vi "Calculate Directions.vi"(8 "error in (no error)":errorcluster, 10 "Heading":T1=enum."Right", 11 "Grassfire in":refnum<class "Grassfire.lvclass">) -> (0 "error out":errorcluster, 2 "Directions":T1[](array[typedef]), 3 "Grassfire out":refnum<class "Grassfire.lvclass">)   [LabVIEW 2019, in "Grassfire.lvclass"]
uses:
  Grassfire.lvclass
  Direction--enum.ctl
  Address/Address.lvclass
  Grassfire.lvclass/Grassfire.ctl
  Node/Node Value.lvclass/Node Value.ctl
  Node/Node Type--enum.ctl
  <userlib>/_OpenG.lib/array/array.llb/Sort 1D Array (I32)__ogtk.vi
  <userlib>/_OpenG.lib/array/array.llb/Reorder 1D Array2 (I16)__ogtk.vi
  Node/Node Value.lvclass
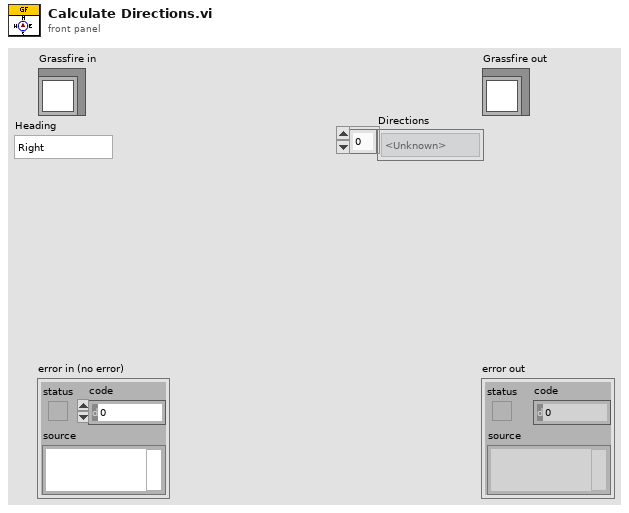
[diagram p1: front panel]
types:
  T1 = typedef "Grassfire.lvclass/Direction--enum.ctl" = enum16{"<Unknown>", "Right", "Down", "Left", "Up"}
  T2 = map{refnum<class "Address.lvclass">, refnum<class "Node Value.lvclass">}
  T3 = typedef "Node Value.lvclass/Node Type--enum.ctl" = enum16{"Empty", "Blocked", "Start", "End", "Path"}
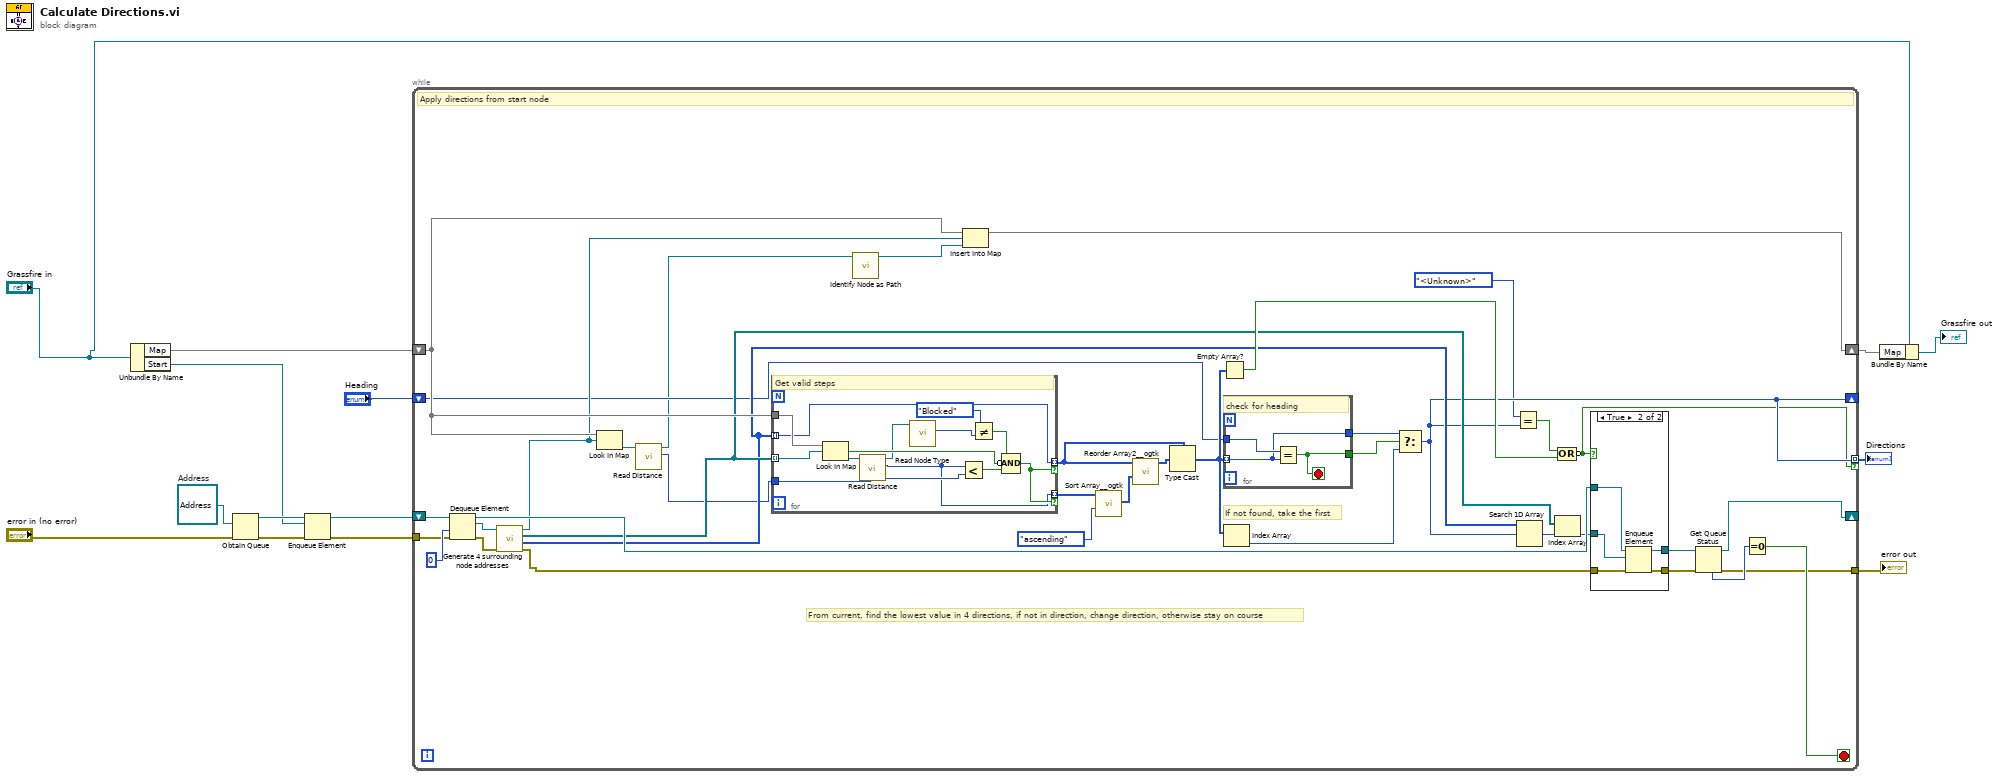
[diagram p0: block diagram]
diagram:
  w1 = refnum<class "Address.lvclass"> refnum  # Address
  n1 = Unbundle By Name("Grassfire in") -> ("Map"=w11:T2, "Start"=w10:refnum<class "Address.lvclass">)
  n2 = Obtain Queue(element data type=w1, error in (no error)="error in (no error)") -> (queue out=w13:refnum<queue>, error out=w14:errorcluster)  [unwired: 3 in, 1 out]
  n3 = Enqueue Element(queue=w13, element=w10, error in (no error)=w14) -> (queue out=w9:refnum<queue>, error out=w8:errorcluster)  [unwired: 1 in, 1 out]
  n4 = while {
    shift-right: [w48] -> w5
    shift-left: w11 -> [w49]
    shift-right: [w47] -> _
    shift-left: w9 -> [w51]
    tunnel: w8 -> [w52]
    tunnel: [w29] -> w7
    shift-right: [w17] -> _
    shift-left: "Heading" -> [w24]
    tunnel: [w17] -> w2 mode=indexing if=w16
    stop <- w46 stop-if-true
    # "If not found, take the first"
    # "From current, find the lowest value in 4 directions, if not in direction, change direction, otherwise stay on course"
    # "Apply directions from start node"
    n5 = Dequeue Element(queue=w51, timeout in ms (-1)=0, error in (no error)=w52) -> (queue out=w50:refnum<queue>, element=w28:refnum<class "Address.lvclass">, error out=w23:errorcluster)  [unwired: 1 out]
    n6 = call "Generate 4 surrounding node addresses.vi"("error in (no error)"=w23, "2D Array in"=w28) -> ("error out"=w22:errorcluster, "Search Directions"=w26:T1[], "4 Surrounding Nodes"=w27:refnum<class "Address.lvclass">[], "2D Array out"=w25:refnum<class "Address.lvclass">)  [unwired: 6 in]
    n7 = Look In Map(map=w49, key=w25) -> (value=w20:refnum<class "Node Value.lvclass">)  [unwired: 1 in, 1 out]
    n8 = call "Read Distance.vi"("Picture Ring in"=w20) -> ("Distance"=w18:i32, "Picture Ring out"=w19:refnum<class "Node Value.lvclass">)  [unwired: 8 in, 1 out]
    n9 = for {
      tunnel: w49 -> [w76]
      tunnel: w27 -> [w75] mode=indexing
      tunnel: [w69] -> w44 mode=indexing if=w73
      tunnel: [w74] -> w40 mode=indexing if=w73
      tunnel: w26 -> [w74] mode=indexing
      tunnel: w18 -> [w71]
      # "Get valid steps"
      n10 = Look In Map(map=w76, key=w75) -> (key not found?=w68:bool, value=w70:refnum<class "Node Value.lvclass">)  [unwired: 1 in]
      n11 = call "Read Distance.vi"("Picture Ring in"=w70) -> ("Distance"=w69:i32, "Picture Ring out"=w67:refnum<class "Node Value.lvclass">)  [unwired: 8 in, 1 out]
      n12 = call "Read Node Type.vi"("Picture Ring in"=w67) -> ("Node Type"=w65:T3)  [unwired: 8 in, 2 out]
      n13 = Less?(x=w69, y=w71) -> (x < y?=w72:bool)
      n14 = Not Equal?(x=Node_Type--enum."Blocked" ("Node Type"), y=w65) -> (x != y?=w64:bool)
      n15 = Compound Arithmetic op=AND(w64, invert w68, w72) -> (w73:bool)
    }
    n16 = call "Identify Node as Path.vi"("Picture Ring in"=w19) -> ("Picture Ring out"=w21:refnum<class "Node Value.lvclass">)  [unwired: 9 in, 1 out]
    n17 = Insert Into Map(map in=w49, key=w25, value=w21) -> (map out=w48:T2)  [unwired: 2 out]
    n18 = call-poly <userlib>:"Sort Array__ogtk.vi"("Order"=enum16{"ascending", "descending"}."ascending", "Array in"=w44) -> ("Sorted Pointers"=w42:i32[])  [unwired: 8 in, 1 out]
    n19 = call-poly <userlib>:"Reorder Array2__ogtk.vi"("indices"=w42, "array"=w40) -> ("reordered array"=w41:i16[])  [unwired: 9 in]
    n20 = Type Cast(type=w40, x=w41) -> (*(type *) &x=w32:T1[])
    n21 = Empty Array?(array=w32) -> (empty?=w38:bool)
    n22 = for {
      tunnel: w32 -> [w62] mode=indexing
      tunnel: w24 -> [w63]
      tunnel: [w62] -> w31
      tunnel: [w61] -> w33
      stop <- w61 stop-if-true
      # "check for heading"
      n23 = Equal?(x=w63, y=w62) -> (x = y?=w61:bool)
    }
    n24 = Index Array(array=w32) -> (element=w30:T1)  [unwired: 1 in]
    n25 = Select(t=w31, s=w33, f=w30) -> (s? t:f=w17:T1)
    n26 = Equal?(x=Direction--enum."<Unknown>" ("Direction"), y=w17) -> (x = y?=w39:bool)
    n27 = Search 1D Array(1D array=w26, element=w17) -> (index of element=w37:i32)  [unwired: 1 in]
    n28 = Index Array(array=w27, index=w37) -> (element=w34:refnum<class "Address.lvclass">)
    n29 = Compound Arithmetic op=OR(w39, w38) -> (invert w16:bool)
    n30 = case shown="True" w16 {
      tunnel: w50 -> [w55 w60]
      tunnel: w22 -> [w54 w59]
      tunnel: [w55 w58] -> w36
      tunnel: [w54 w57] -> w35
      tunnel: w34 -> [_ w56]
      frame False {
      }
      frame True {
        n31 = Enqueue Element(queue=w60, element=w56, error in (no error)=w59) -> (queue out=w58:refnum<queue>, error out=w57:errorcluster)  [unwired: 1 in, 1 out]
      }
    }
    n32 = Get Queue Status(queue=w36, error in (no error)=w35) -> (queue out=w47:refnum<queue>, error out=w29:errorcluster, # elements in queue=w45:i32)  [unwired: 1 in, 5 out]
    n33 = Equal To 0?(x=w45) -> (x = 0?=w46:bool)
  }
  "error out" <- w7
  "Directions" <- w2
  n34 = Bundle By Name(cluster="Grassfire in", "Map"=w5) -> (→"Grassfire out":refnum<class "Grassfire.lvclass">)
